vi "Compute DistanceToTarget2.vi"(10 "Normalized Rect":T1, 11 "Camera Type":T2) -> (3 "Distance (ft)":dbl)   [LabVIEW 2025]
doc: "Using the camera lens information and the real world size of the target, use trig and ratios to determine the distance to the target. Also returns the location relative to the image center in a (-1 , 1) coordinate system that may be useful for steering the robot."
uses:
  Camera Types.ctl
panel:
  # "Axis 206\nAxis M1011\nAxis M1013\nMS HD3000 square\nMS HD 3000 640x480"
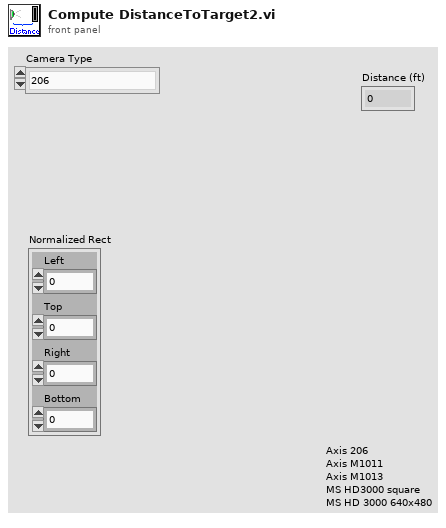
[diagram p1: front panel]
types:
  T1 = cluster{"Left":dbl, "Top":dbl, "Right":dbl, "Bottom":dbl}
  T2 = typedef "Camera Types.ctl" = enum16{"206", "1011", "1013", "MS HD3000 square", "MS HD3000 640x480"}
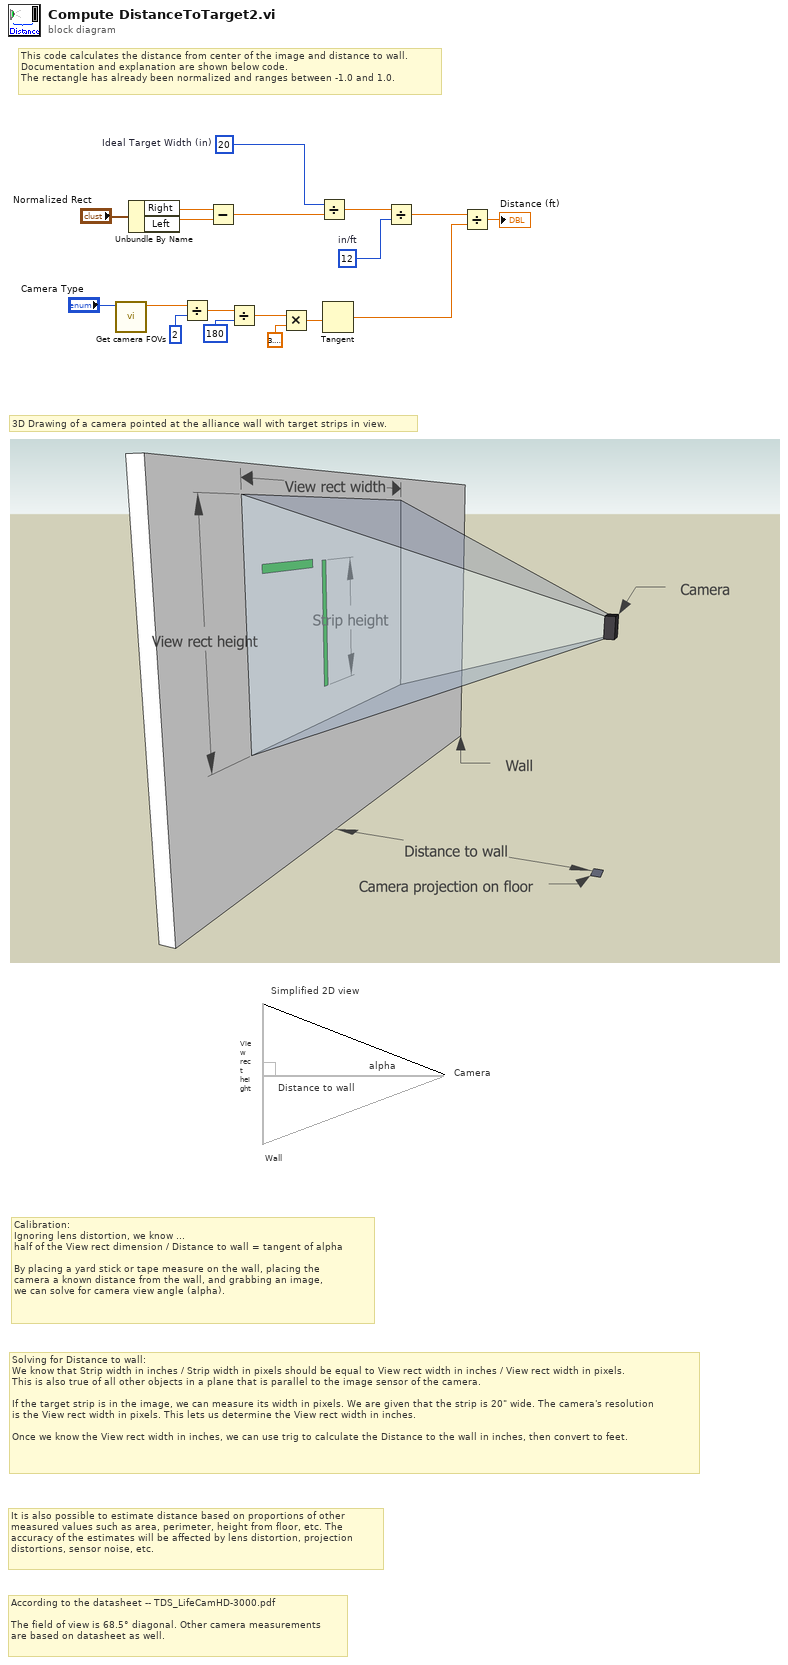
[diagram p0: block diagram]
diagram:
  w1 = 20  # Ideal Target Width (in)
  w11 = 12  # in/ft
  # "It is also possible to estimate distance based on proportions of other\nmeasured values such as area, perimeter, height from floor, etc. The\naccuracy of the estimates will be affected by lens distortion, projection\ndistortions, sensor noise, etc."
  # "According to the datasheet -- TDS_LifeCamHD-3000.pdf\n\nThe field of view is 68.5° diagonal. Other camera measurements\nare based on datasheet as well."
  # "Wall"
  # "Camera"
  # "Simplified 2D view"
  # "Solving for Distance to wall:\nWe know that Strip width in inches / Strip width in pixels should be equal to View rect width in inches / View rect width in pixels.\nThis is also true of all other objects in a plane that is parallel to the image sensor of the camera.\n\nIf the target strip is in the image, we can measure its width in pixels. We are given that the strip is 20\" wide. The camera's resolution\nis the View rect width in pixels. This lets us determine the View rect width in inches.\n\nOnce we know the View rect width in inches, we can use trig to calculate the Distance to the wall in inches, then convert to feet."
  # "3D Drawing of a camera pointed at the alliance wall with target strips in view."
  # "Distance to wall"
  # "View rect height"
  # "alpha"
  # "Calibration:\nIgnoring lens distortion, we know ...\nhalf of the View rect dimension / Distance to wall = tangent of alpha\n\nBy placing a yard stick or tape measure on the wall, placing the\ncamera a known distance from the wall, and grabbing an image,\nwe can solve for camera view angle (alpha)."
  # "This code calculates the distance from center of the image and distance to wall.\nDocumentation and explanation are shown below code.\nThe rectangle has already been normalized and ranges between -1.0 and 1.0."
  n1 = call "Get camera FOVs.vi"("Camera Type"="Camera Type") -> ("FOV"=w3:dbl)  [unwired: 9 in, 1 out]
  n2 = Unbundle By Name("Normalized Rect") -> ("Right"=w8:dbl, "Left"=w7:dbl)
  n3 = Divide(x=w3, y=2) -> (x/y=w15:dbl)
  n4 = Subtract(x=w8, y=w7) -> (x-y=w6:dbl)
  n5 = Divide(x=w15, y=180) -> (x/y=w14:dbl)
  n6 = Multiply(x=w14, y=3.141592653589793) -> (x*y=w16:dbl)
  n7 = Divide(x=w1, y=w6) -> (x/y=w5:dbl)
  n8 = Tangent(1:w16) -> (0:w10:dbl)
  n9 = Divide(x=w5, y=w11) -> (x/y=w4:dbl)
  n10 = Divide(x=w4, y=w10) -> (x/y=→"Distance (ft)":dbl)
